vi "Set Display Infos.vi"(5 "Direction info in":string, 7 "Boost info in":string, 11 "Game Board in":refnum<class "Game Board.lvclass">) -> ()   [LabVIEW 2024, in "Game Board.lvclass"]
doc: "MIT Licence\nCopyright (c) 2024 David Grollier"
uses:
  Game Board.lvclass
  Game Board.lvclass/Game Board.ctl
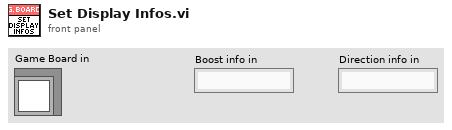
[diagram p1: front panel]
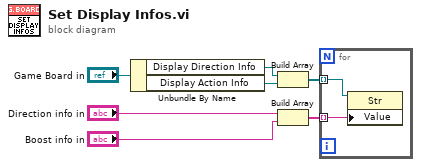
[diagram p0: block diagram]
diagram:
  n1 = Unbundle By Name("Game Board in") -> ("Display Direction Info"=w6:refnum<vi>, "Display Action Info"=w5:refnum<vi>)
  n2 = Build Array(w6, w5) -> (w2:refnum<vi>[])
  n3 = Build Array("Direction info in", "Boost info in") -> (w1:string[])
  n4 = for {
    tunnel: w2 -> [w9] mode=indexing
    tunnel: w1 -> [w8] mode=indexing
    n5 = property class="Str"(reference=w9, "Value"=w8) -> ()  [unwired: 1 in, 2 out]
  }
